vi "from string.vi"(8 "error in":errorcluster, 9 "data":string, 10 "version":string, 11 "TDMS datalogger configuration in":refnum<class "TDMS datalogger configuration.lvclass">) -> (0 "error out":errorcluster, 3 "TDMS datalogger configuration out":refnum<class "TDMS datalogger configuration.lvclass">)   [LabVIEW 2013, in "TDMS datalogger configuration.lvclass"]
doc: "Provides an interface for loading a module configuration from a file or other serialized data source. It is recommended that all children of this class store data in two sets--data required for its own initialization, and any data required for parent initialization--and that each implementation uses the <b>Call Parent Method</b> primitive to de-serialize parent information. As a result, it is expected that every module configuration class calls <b>component configuration.lvclass:From String.vi</b>."
uses:
  TDMS datalogger configuration.lvclass
  <vilib>/NI/Tag Bus Module Framework/channel/TBM channel.lvclass
  <vilib>/NI/Tag Bus Module Framework/module configuration/TBM module configuration.lvclass
  TDMS datalogger configuration.lvclass/TDMS datalogger configuration.ctl
  <vilib>/NI/Tag Bus Module Framework/root configuration/TBM configuration.lvclass
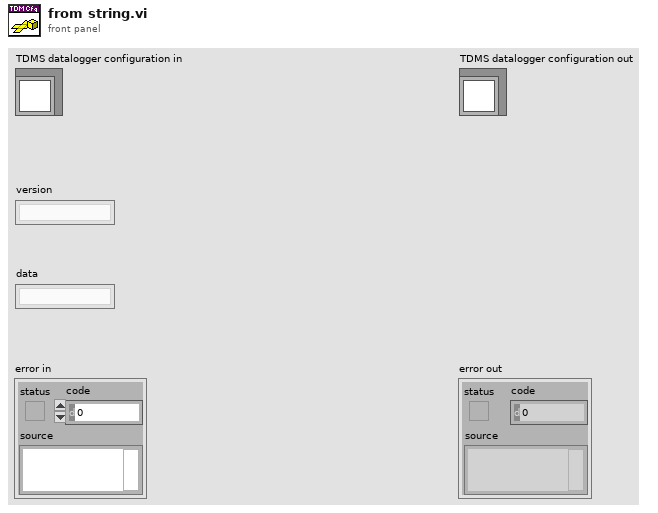
[diagram p1: front panel]
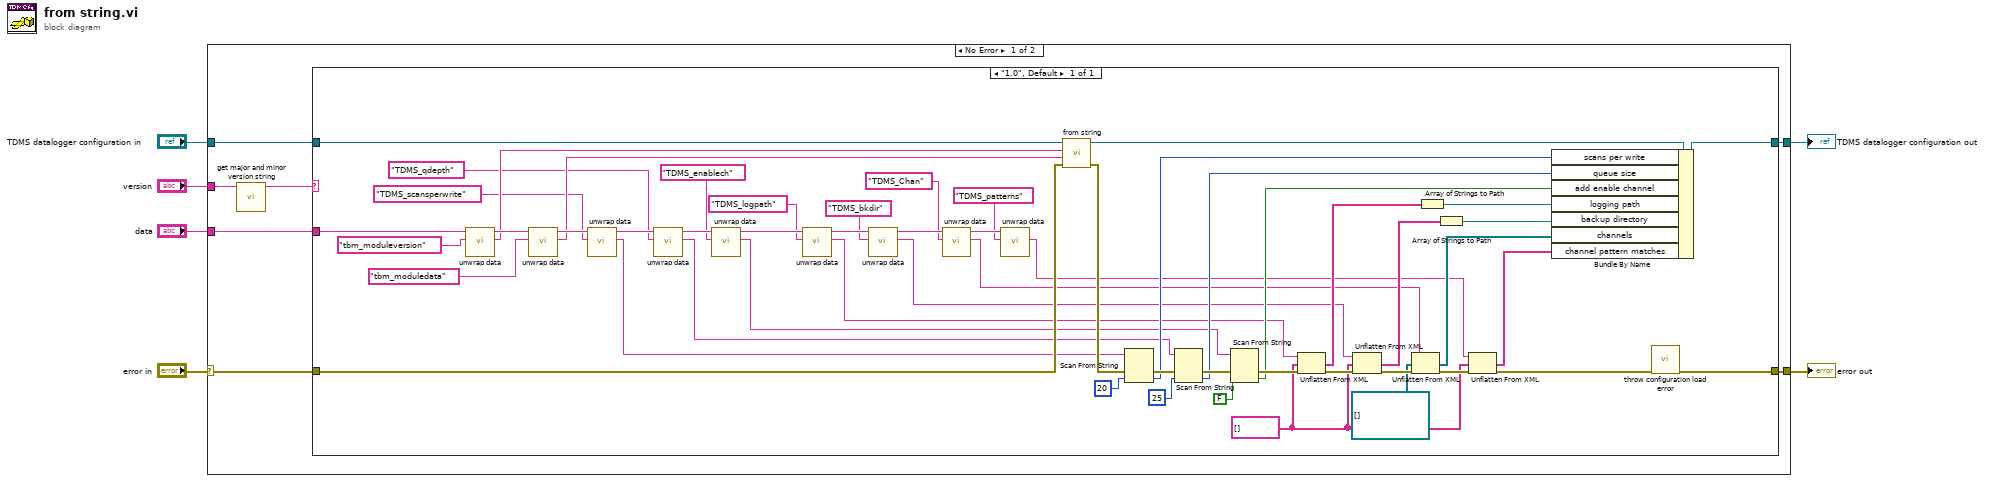
[diagram p0: block diagram]
diagram:
  n1 = case shown="No Error" "error in" {
    selector: "error in" -> [w7 w69]
    tunnel: "data" -> [w13 _]
    tunnel: "TDMS datalogger configuration in" -> [w12 w68]
    tunnel: [w11 w68] -> w5
    tunnel: [w10 w69] -> w4
    tunnel: "version" -> [w9 _]
    frame No Error {
      n2 = call <vilib>:"get major and minor version string.vi"("full version"=w9) -> ("major.minor version"=w8:string)  [unwired: 10 in]
      n3 = case shown="\"1.0\", Default" w8 {
        tunnel: w13 -> [w48]
        tunnel: w7 -> [w64]
        tunnel: w12 -> [w67]
        tunnel: [w66] -> w11
        tunnel: [w21] -> w10
        frame "1.0", Default {
          w16 = string[] [] ("array of strings")
          n4 = call <vilib>:"unwrap data.vi"("identifier"="tbm_moduleversion" ("additional identifier"), "data to unwrap"=w48) -> ("unwrapped data"=w47:string, "remaining string"=w54:string)  [unwired: 8 in]
          n5 = call <vilib>:"unwrap data.vi"("identifier"="tbm_moduledata" ("additional identifier"), "data to unwrap"=w54) -> ("unwrapped data"=w46:string, "remaining string"=w51:string)  [unwired: 8 in]
          n6 = call <vilib>:"unwrap data.vi"("identifier"="TDMS_scansperwrite" ("additional identifier"), "data to unwrap"=w51) -> ("unwrapped data"=w32:string, "remaining string"=w50:string)  [unwired: 8 in]
          n7 = call <vilib>:"unwrap data.vi"("identifier"="TDMS_qdepth" ("additional identifier"), "data to unwrap"=w50) -> ("unwrapped data"=w30:string, "remaining string"=w49:string)  [unwired: 8 in]
          n8 = call <vilib>:"unwrap data.vi"("identifier"="TDMS_enablech" ("additional identifier"), "data to unwrap"=w49) -> ("unwrapped data"=w28:string, "remaining string"=w36:string)  [unwired: 8 in]
          n9 = call <vilib>:"unwrap data.vi"("identifier"="TDMS_logpath" ("additional identifier"), "data to unwrap"=w36) -> ("unwrapped data"=w26:string, "remaining string"=w35:string)  [unwired: 8 in]
          n10 = call <vilib>:"unwrap data.vi"("identifier"="TDMS_bkdir" ("additional identifier"), "data to unwrap"=w35) -> ("unwrapped data"=w25:string, "remaining string"=w34:string)  [unwired: 8 in]
          n11 = call <vilib>:"unwrap data.vi"("identifier"="TDMS_Chan" ("additional identifier"), "data to unwrap"=w34) -> ("unwrapped data"=w24:string, "remaining string"=w20:string)  [unwired: 8 in]
          n12 = call <vilib>:"unwrap data.vi"("identifier"="TDMS_patterns", "data to unwrap"=w20) -> ("unwrapped data"=w15:string)  [unwired: 8 in, 1 out]
          n13 = call-parent "from string.vi"("error in"=w64, "data"=w46, "version"=w47, "module configuration in"=w67) -> ("error out"=w65:errorcluster, "module configuration out"=w63:refnum<class "TDMS datalogger configuration.lvclass">)  [unwired: 6 in]
          n14 = Scan From String(input string=w32, error in=w65, default 1=20 ("scans per write")) -> (error out=w43:errorcluster, output 1=w37:i32)  [unwired: 2 in, 2 out]
          n15 = Scan From String(input string=w30, error in=w43, default 1=25 ("queue size")) -> (error out=w44:errorcluster, output 1=w39:i32)  [unwired: 2 in, 2 out]
          n16 = Scan From String(input string=w28, error in=w44, default 1=FALSE ("add enable channel")) -> (error out=w45:errorcluster, output 1=w41:bool)  [unwired: 2 in, 2 out]
          n17 = Unflatten From XML(xml string=w26, type=w16, error in (no error)=w45) -> (value=w55:string[], error out=w59:errorcluster)
          n18 = Unflatten From XML(xml string=w25, type=w16, error in (no error)=w59) -> (value=w56:string[], error out=w60:errorcluster)
          n19 = Unflatten From XML(xml string=w24, type=refnum<class "TBM channel.lvclass">[] [] ("channels"), error in (no error)=w60) -> (value=w57:refnum<class "TBM channel.lvclass">[], error out=w18:errorcluster)
          n20 = Array of Strings to Path(0:w55) -> (2:w62:path)  [unwired: 1 in]
          n21 = Array of Strings to Path(0:w56) -> (2:w61:path)  [unwired: 1 in]
          n22 = Unflatten From XML(xml string=w15, type=w16, error in (no error)=w18) -> (value=w14:string[], error out=w17:errorcluster)
          n23 = Bundle By Name(cluster=w63, "scans per write"=w37, "queue size"=w39, "add enable channel"=w41, "logging path"=w62, "backup directory"=w61, "channels"=w57, "channel pattern matches"=w14) -> (w66:refnum<class "TDMS datalogger configuration.lvclass">)
          n24 = call <vilib>:"throw configuration load error.vi"("error in"=w17) -> ("error out"=w21:errorcluster)  [unwired: 10 in]
        }
      }
    }
    frame Error {
    }
  }
  "error out" <- w4
  "TDMS datalogger configuration out" <- w5
